vi "robot_position_test.vi"() -> ()   [LabVIEW 2009]
uses:
  OGRE/nick/FPGA/behaviors/driveable paths/test variable.vi
panel:
  in  "Iterations":i32
  out "Y positions":i16[](array[numeric])
  out "x positions":i16[](array[numeric])
  out "XY Graph":cluster{"Y":dbl[], "Y":dbl[]}[](graph)
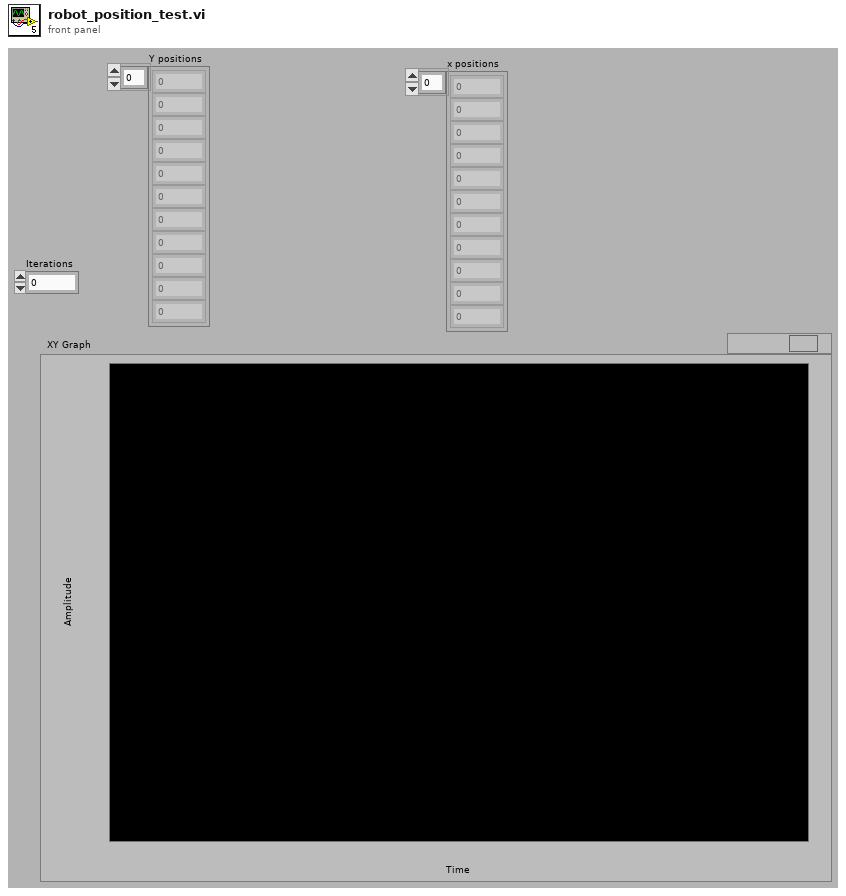
[diagram p1: front panel]
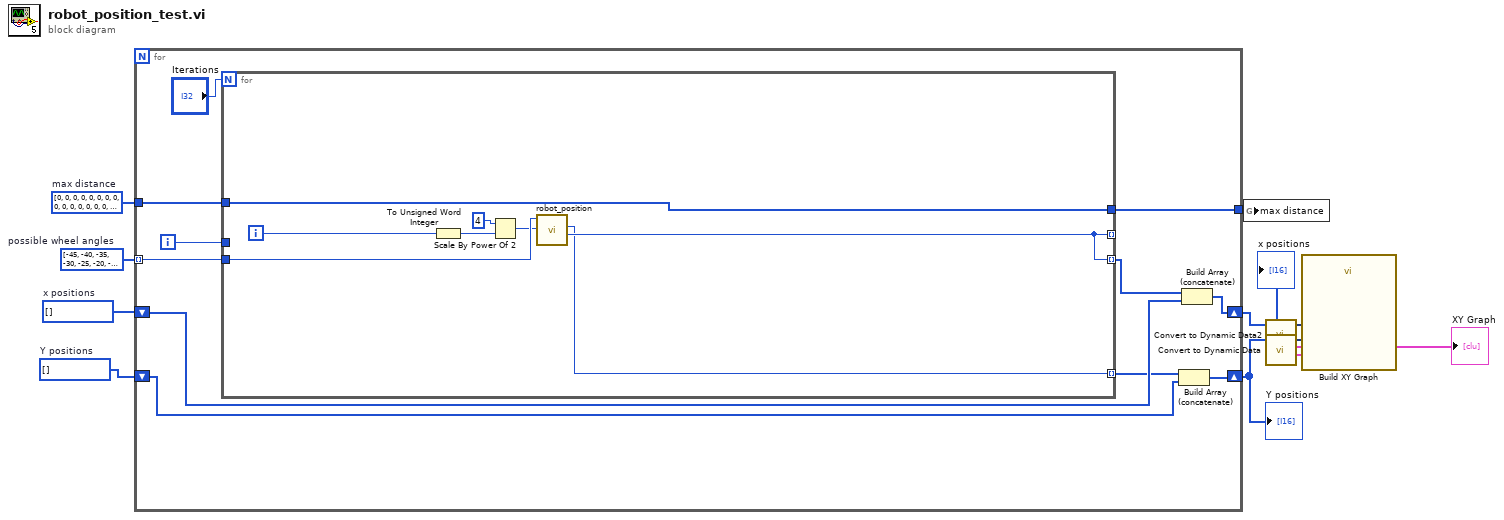
[diagram p0: block diagram]
diagram:
  w5 = i8[] []  # Y positions
  w6 = i8[] []  # x positions
  w8 = i8[] [-45, -40, -35, -30, -25, -20, -15, -10, -5, 0, 5, 10, 15, 20, 25, 30, 35, 40, 45]  # possible wheel angles
  w9 = i16[] [0, 0, 0, 0, 0, 0, 0, 0, 0, 0, 0, 0, 0, 0, 0, 0, 0, 0, 0]  # max distance
  n1 = for {
    tunnel: w9 -> [w21]
    tunnel: w8 -> [w12] mode=indexing
    tunnel: [w19] -> w7
    shift-right: [w16] -> w2
    shift-left: w6 -> [w17]
    shift-right: [w15] -> w4
    shift-left: w5 -> [w13]
    i -> [w20]
    n2 = for {
      N: "Iterations" -> [_]
      tunnel: w21 -> [w25]
      tunnel: [w25] -> w19
      tunnel: w20 -> [_]
      tunnel: w12 -> [w28]
      tunnel: [w24] -> _ mode=indexing
      tunnel: [w24] -> w18 mode=indexing
      tunnel: [w23] -> w14 mode=indexing
      i -> [w29]
      n3 = To Unsigned Word Integer(number=w29) -> (unsigned 16bit integer=w26:u16)
      n4 = Scale By Power Of 2(n=u16 4, x=w26) -> (x*2^n=w22:u16)
      n5 = call "robot_position.vi"("Distance Along Arc"=w22, "Wheel Angle"=w28) -> ("New X Position"=w24:i8, "New Y Position"=w23:i8)  [unwired: 7 in, 1 out]
    }
    n6 = Build Array (concatenate)(w14, w13) -> (w15:i8[])
    n7 = Build Array (concatenate)(w18, w17) -> (w16:i8[])
  }
  "x positions" <- w2
  "Y positions" <- w4
  n8 = global write "test variable.vi" "max distance"(w7) -> ()
  n9 = call "Convert to Dynamic Data2"("Array"=w2) -> ("Dynamic Data Type"=w1:dynamicdata)  [unwired: 3 in]
  n10 = call "Convert to Dynamic Data"("Array"=w4) -> ("Dynamic Data Type"=w3:dynamicdata)  [unwired: 3 in]
  n11 = call "Build XY Graph"("Y Input"=w3, "X Input"=w1) -> ("XY Graph"=→"XY Graph":cluster{"Y":dbl[], "Y":dbl[]}[])  [unwired: 8 in, 1 out]
